vi "Mask Payload.vi"(7 "mask":u8[](array[numeric]), 10 "Input":u8[](array[numeric])) -> (2 "Output":u8[](array[numeric]))   [LabVIEW 2013, in "Connection.WS_GOSPL.lvlib" / "Connection.WS.lvclass"]
uses:
  Connection.WS.lvclass
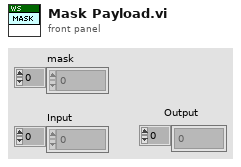
[diagram p1: front panel]
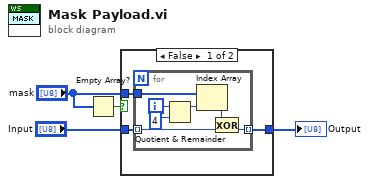
[diagram p0: block diagram]
diagram:
  n1 = Empty Array?(array="mask") -> (empty?=w2:bool)
  n2 = case shown="False" w2 {
    tunnel: [w7 w15] -> w4
    tunnel: "Input" -> [w6 w15]
    tunnel: "mask" -> [w5 _]
    frame False {
      n3 = for {
        tunnel: w6 -> [w14] mode=indexing
        tunnel: w5 -> [w10]
        tunnel: [w8] -> w7 mode=indexing
        i -> [w13]
        n4 = Quotient & Remainder(x=w13, y=4) -> (x-y*floor(x/y)=w11:i32)  [unwired: 1 out]
        n5 = Index Array(array=w10, index=w11) -> (element=w9:u8)
        n6 = Exclusive Or(1:w14, 2:w9) -> (0:w8:u8)
      }
    }
    frame True {
    }
  }
  "Output" <- w4
